vi "RenameFiles.vi"() -> ()   [LabVIEW 2014]
panel:
  out "Array 2":string[](array[string])
  out "Array":string[](array[string])
  in  "pattern":string
  in  "Folder Path":path
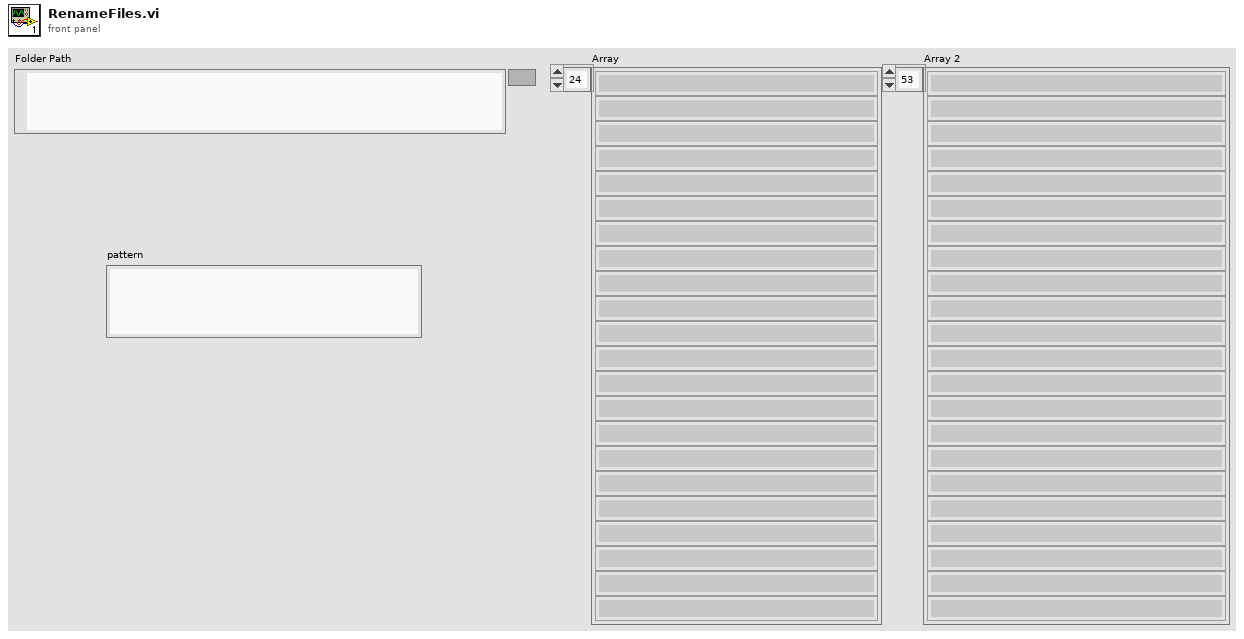
[diagram p1: front panel]
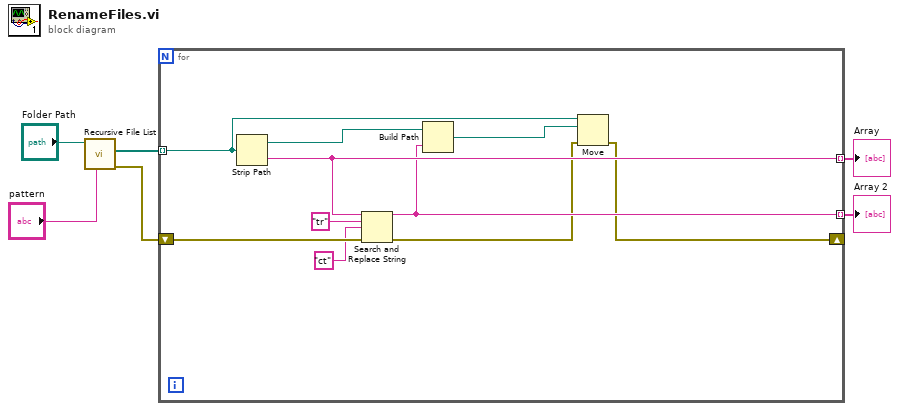
[diagram p0: block diagram]
diagram:
  n1 = call <vilib>:"Recursive File List.vi"("pattern"="pattern", "Folder Path"="Folder Path") -> ("error out"=w1:errorcluster, "All Files in Dir"=w4:path[])  [unwired: 5 in, 3 out]
  n2 = for {
    tunnel: w4 -> [w13] mode=indexing
    tunnel: [w12] -> w3 mode=indexing
    tunnel: [w10] -> w2 mode=indexing
    shift-right: [w7] -> _
    shift-left: w1 -> [w15]
    n3 = Strip Path(path=w13) -> (stripped path=w11:path, name=w12:string)
    n4 = Search and Replace String(input string=w12, search string="tr", replace string="ct" ("replace string (\"\")"), error in=w15) -> (result string=w10:string, error out=w8:errorcluster)  [unwired: 4 in, 2 out]
    n5 = Build Path(base path=w11, name or relative path=w10) -> (appended path=w9:path)
    n6 = Move(source path=w13, error in=w8, 10:w9) -> (error out=w7:errorcluster)  [unwired: 2 in, 2 out]
  }
  "Array" <- w3
  "Array 2" <- w2
